vi "Pigeon2 Robot Centric.vi"(10 "Robot Centric Velocities":T1) -> (3 "Field Centric Velocities":T1)   [LabVIEW 2025]
uses:
  Type Definitions/Data/Robot Velocities.ctl
  <vilib>/Analysis/coordinate.llb/Angle Units.ctl
  <vilib>/Analysis/coordinate.llb/Wrap Angle (scalar).vi
  Robot Code/Framework/Robot Global Data.vi
  <vilib>/Analysis/NI_AAL_Angle.lvlib
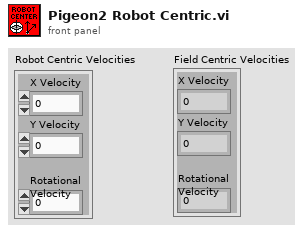
[diagram p1: front panel]
types:
  T1 = typedef "Robot Velocities.ctl" = cluster{"X Velocity":dbl, "Y Velocity":dbl, "Rotational \nVelocity":dbl}
  T2 = typedef "NI_AAL_Angle.lvlib/Angle Units.ctl" = i32
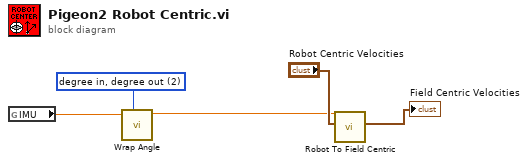
[diagram p0: block diagram]
diagram:
  w3 = T2 2 items=["radian in, radian out", "radian in, degree out", "degree in, degree out", "degree in, radian out"] ("angle units")
  n1 = global read "Robot Global Data.vi" "IMU"() -> (w1:dbl)
  n2 = call-poly <vilib>:"Wrap Angle.vi"("angle units"=w3, "angle in"=w1) -> ("angle out"=w2:dbl)  [unwired: 8 in, 1 out]
  n3 = call "Robot To Field Centric.vi"("Robot Centric Velocities"="Robot Centric Velocities", "IMU Value (offset)"=w2) -> ("Field Centric Velocities"=→"Field Centric Velocities":T1)  [unwired: 8 in, 1 out]
